vi "Ardunio Analog Read.vi"() -> ()   [LabVIEW 2022 SP3]
uses:
  <vilib>/MakerHub/LINX/Public/Peripherals/Analog/Analog Read N Chans.vi
  <vilib>/MakerHub/LINX/Private/Local IO/LinxAnalogRead.vi
  <vilib>/MakerHub/LINX/Public/Utilities/Check Channel.vi
  <vilib>/MakerHub/LINX/Public/Utilities/Open Serial.vi
  <vilib>/MakerHub/LINX/Private/Utilties/Generate Error.vi
  <vilib>/MakerHub/LINX/LMH-LINX.lvlib
panel:
  out "Exit?":bool
  in  "stop":bool
  in  "Tab Control":enum32{"Main", "Graphs"}(tab)
  in  "start":bool
  out "Device Name":string
  in  "Tab Control 2":T1(tab)
  out "Waveform Chart":dbl(graph)
  in  "Radio Buttons":T2(radio)
  # "Gerilim"
  # "s1cakl1k"
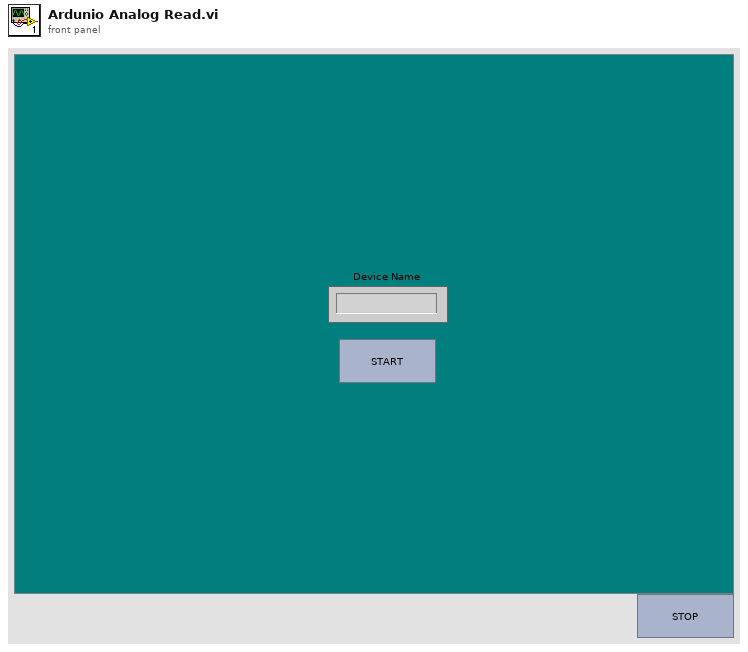
[diagram p1: front panel]
types:
  T1 = enum32{"Voltage Measurement Graph", "Temperature Measurement Graph", "DC current measurement Graph"}
  T2 = enum32{"Voltage Measurement Graph", "Temperature Measurement Graph", "DC current measurement"}
  T3 = enum16{"initialize", "AnalogRead", "VoltageGraph", "TemperatureGraph", "CurrentGraph"}
  T4 = cluster{"Voltage":dbl, "Temperature":dbl, "Current":dbl}
  T5 = enum16{"initialize", "Wait for Event", "start", "stop"}
  T6 = typedef "LMH-LINX.lvlib/LINX Ref.ctl" = cluster{"IO":T7, "Interface":T8, "LINX Device Config":T9}
  T7 = typedef "LMH-LINX.lvlib/Platform.ctl" = enum16{"Remote", "Local"}
  T8 = typedef "LMH-LINX.lvlib/Interface.ctl" = enum16{"Serial", "TCP"}
  T9 = typedef "LMH-LINX.lvlib/Device.lvlib/LINX Device Config.ctl" = cluster{"Interface":T8, "COM Port":refnum<visa-resource-name>, "TCP Configuration":T10, "Device Family":u8, "Device ID":u8, "Device Name":string, "TCP Ref":refnum<k5>, "Channels":T11}
  T10 = typedef "LMH-LINX.lvlib/Device.lvlib/TCP Config.ctl" = cluster{"IP Address":string, "Port":u16}
  T11 = typedef "LMH-LINX.lvlib/Channels.ctl" = cluster{"DI":u8[], "DO":u8[], "AI":u8[], "AO":u8[], "PWM":u8[], "QE":u8[], "UART":u8[], "I2C 2":u8[], "SPI":u8[], "CAN":u8[], "Servo":u8[], "AI Ref (V)":dbl, "AI Resolution (Bits)":u8, "AO Ref (V)":dbl, "AO Resolution (Bits)":u8}
  T12 = cluster{"Voltages[0]":dbl, "Voltages[1]":dbl, "Voltages[2]":dbl}
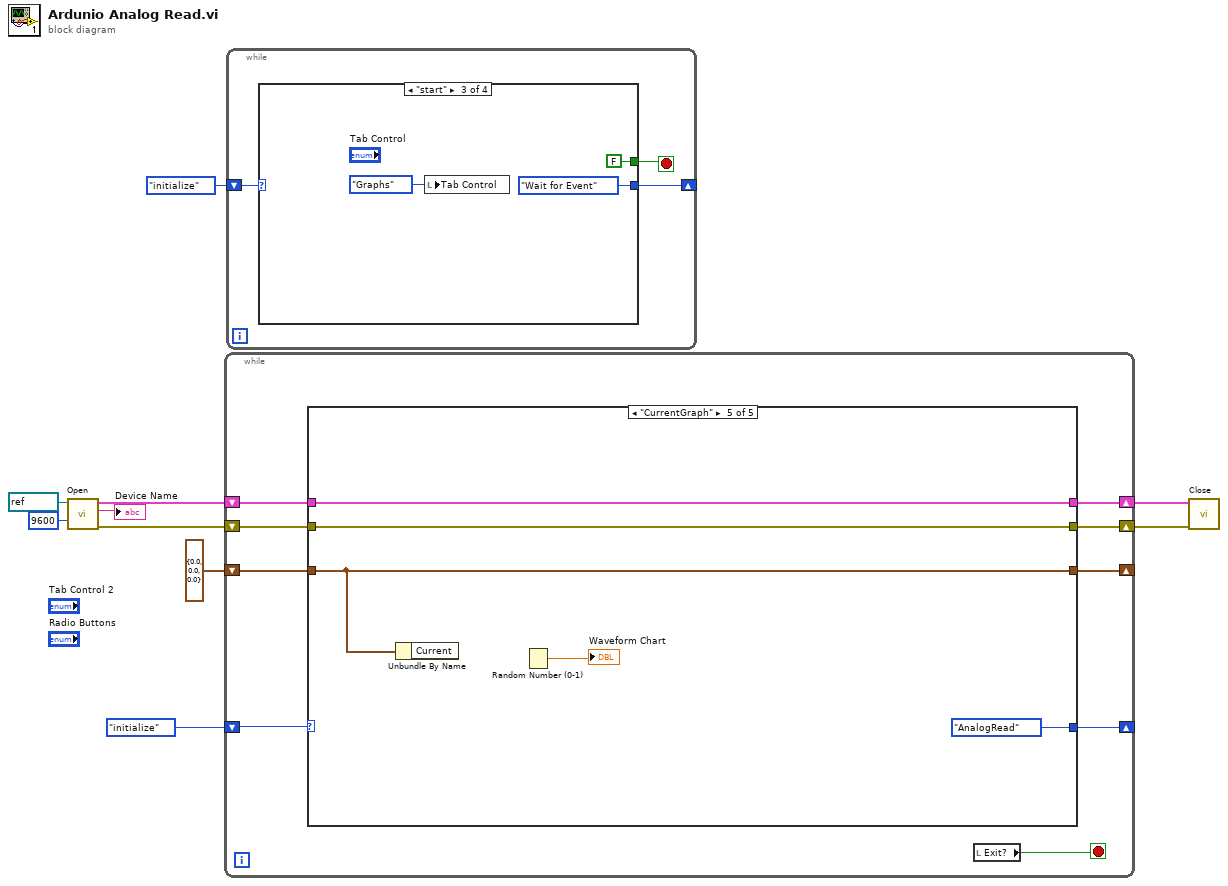
[diagram p0: block diagram]
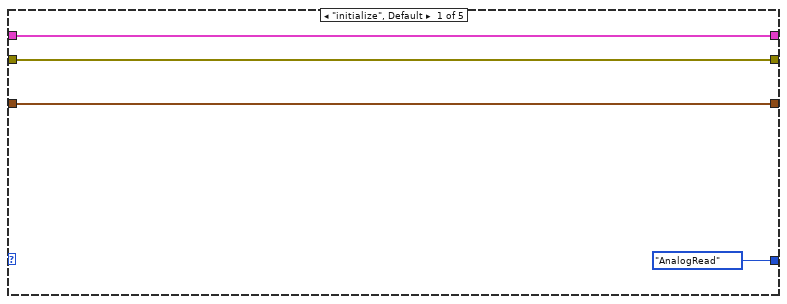
[diagram p2: hidden frame]
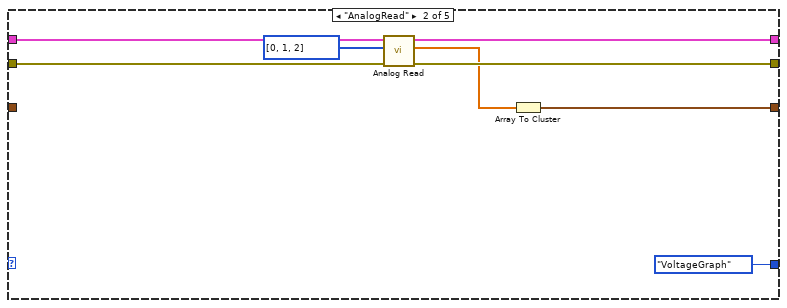
[diagram p3: hidden frame]
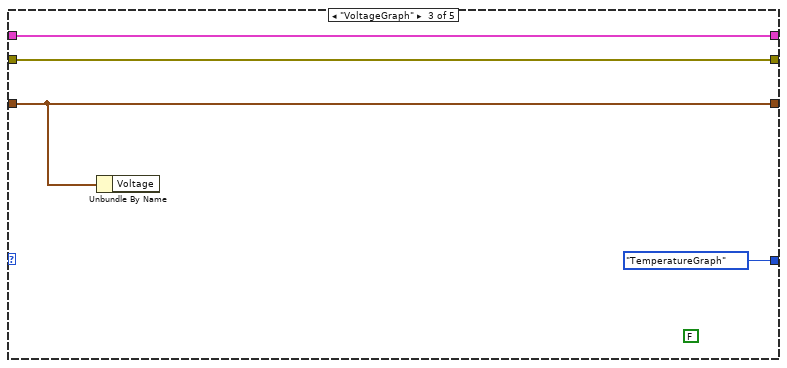
[diagram p4: hidden frame]
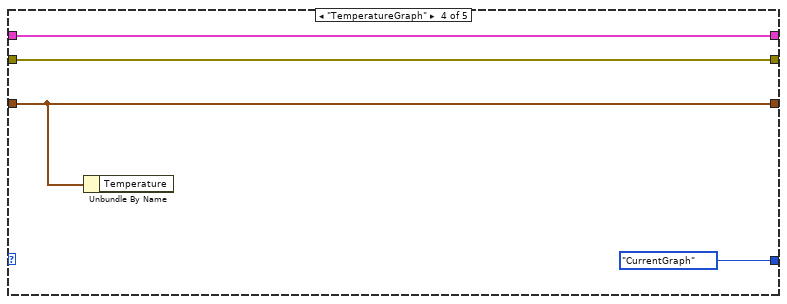
[diagram p5: hidden frame]
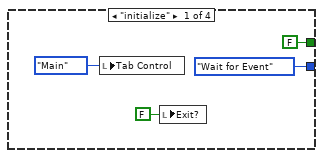
[diagram p6: hidden frame]
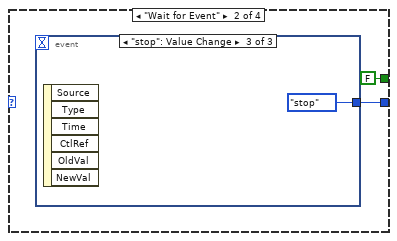
[diagram p7: hidden frame]
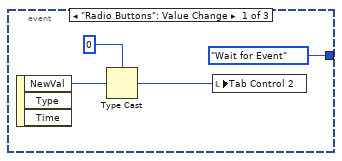
[diagram p8: hidden frame]
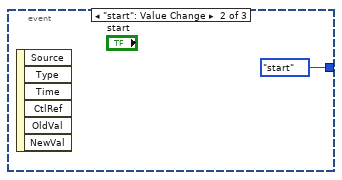
[diagram p9: hidden frame]
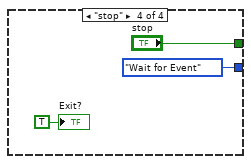
[diagram p10: hidden frame]
diagram:
  n1 = call-poly <vilib>:"Open.vi"("Baud Rate Override"=u32 9600, "Serial Port"=refnum<visa-resource-name> "N/A") -> ("Error Out"=w7:errorcluster, "Device Name"=→"Device Name":string, "LINX Resource"=w5:T6)  [unwired: 7 in]
  n2 = while {
    shift-right: [w12] -> _
    shift-left: T3."initialize" -> [w19]
    shift-right: [w16] -> w4
    shift-left: w5 -> [w17]
    shift-right: [w18] -> w6
    shift-left: w7 -> [w15]
    shift-right: [w14] -> _
    shift-left: T4 {"Voltage"=0.0, "Temperature"=0.0, "Current"=0.0} ("Voltages") -> [w13]
    stop <- w11 stop-if-true
    n3 = case shown="\"CurrentGraph\"" w19 {
      tunnel: w15 -> [w22 w30 w34 w38 w43]
      tunnel: [w22 w29 w34 w38 w43] -> w18
      tunnel: w17 -> [w23 w31 w35 w39 w44]
      tunnel: [w23 w28 w35 w39 w44] -> w16
      tunnel: [w21 w26 w33 w37 w42] -> w14
      tunnel: w13 -> [w21 _ w33 w37 w42]
      tunnel: [T3."AnalogRead" T3."VoltageGraph" T3."TemperatureGraph" T3."CurrentGraph" T3."AnalogRead"] -> w12
      frame "initialize", Default {
      }
      frame "AnalogRead" {
        n4 = call-poly <vilib>:"Analog Read.vi"("Error In"=w30, "AI Channel(s)"=u8[] [0, 1, 2], "LINX Resource"=w31) -> ("Error Out"=w29:errorcluster, "Voltages"=w25:dbl[], "LINX Resource"=w28:T6)  [unwired: 5 in, 1 out]
        n5 = Array To Cluster(array=w25) -> (cluster=w26:T12)
      }
      frame "VoltageGraph" {
        (unwired) FALSE
        n6 = Unbundle By Name(w33) -> ()  [unwired: 1 out]
      }
      frame "TemperatureGraph" {
        n7 = Unbundle By Name(w37) -> ()  [unwired: 1 out]
      }
      frame "CurrentGraph" {
        n8 = Unbundle By Name(w42) -> ()  [unwired: 1 out]
        n9 = Random Number (0-1)() -> (number: 0 to 1=→"Waveform Chart":dbl)
      }
    }
    n10 = local read "Exit?"() -> (w11:bool)
  }
  n11 = while {
    shift-right: [w46] -> _
    shift-left: T5."initialize" -> [w47]
    stop <- w45 stop-if-true
    n12 = case shown="\"start\"" w47 {
      tunnel: [T5."Wait for Event" w53 T5."Wait for Event" T5."Wait for Event"] -> w46
      tunnel: [FALSE ("stop") FALSE ("stop") FALSE ("stop") "stop"] -> w45
      frame "initialize" {
        n13 = local write "Tab Control"(enum32{"Main", "Graphs"}."Main" ("Tab Control")) -> ()
        n14 = local write "Exit?"(FALSE ("Exit?")) -> ()
      }
      frame "Wait for Event" {
        n15 = event shown="[2] \"stop\": Value Change" {
          selector: _ -> [_ _ _]
          dyn-events: _ -> [_ _ _]
          timeout: _ -> [_ _ _]
          tunnel: [T5."Wait for Event" T5."start" T5."stop"] -> w53
          event "Radio Buttons": Value Change {
            n16 = event-data() -> ("NewVal"=w57:T2)  [unwired: 1 in, 2 out]
            n17 = Type Cast(type=0, x=w57) -> (*(type *) &x=w56:i32)
            n18 = local write "Tab Control 2"(w56) -> ()
          }
          event "start": Value Change {
            n19 = event-data() -> ()  [unwired: 1 in, 6 out]
          }
          event "stop": Value Change {
            n20 = event-data() -> ()  [unwired: 1 in, 6 out]
          }
        }
      }
      frame "start" {
        n21 = local write "Tab Control"(enum32{"Main", "Graphs"}."Graphs" ("Tab Control")) -> ()
      }
      frame "stop" {
        "Exit?" <- TRUE ("Exit?")
      }
    }
  }
  n22 = call <vilib>:"Close.vi"("Error In"=w6, "LINX Resource"=w4) -> ()  [unwired: 9 in, 1 out]
